vi "Initialize.vi"(8 "Error In":errorcluster, 9 "timeout in ms (-1)":i32=-1, 10 "WaitOnReply":bool, 11 "Payload":variant) -> (0 "error out":errorcluster, 2 "Reply":variant)   [LabVIEW 2017, in "ErrorHandler.lvlib"]
uses:
  ErrorHandler.lvlib
  States_FGVQ.ctl
  MessageData.ctl
  States_Module.ctl
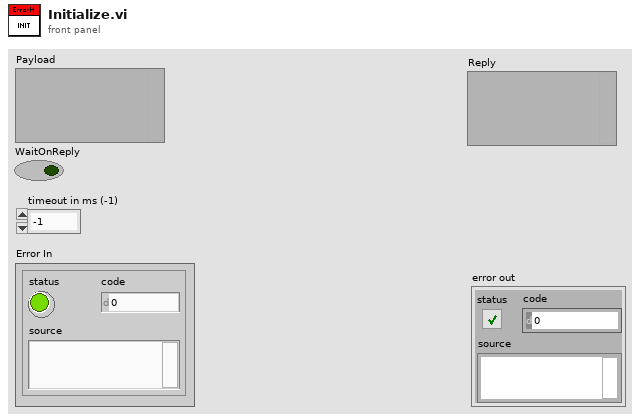
[diagram p1: front panel]
types:
  T1 = typedef "ErrorHandler.lvlib/States_Module.ctl" = enum16{"Error", "DoSomething", "Shutdown", "Initialize"}
  T2 = typedef "ErrorHandler.lvlib/MessageData.ctl" = cluster{"State":T1, "Payload":variant, "WaitOnReply":bool, "ReplyNotif":refnum<notifier>}
  T3 = typedef "ErrorHandler.lvlib/States_FGVQ.ctl" = enum16{"Get", "Shutdown", "Initialize"}
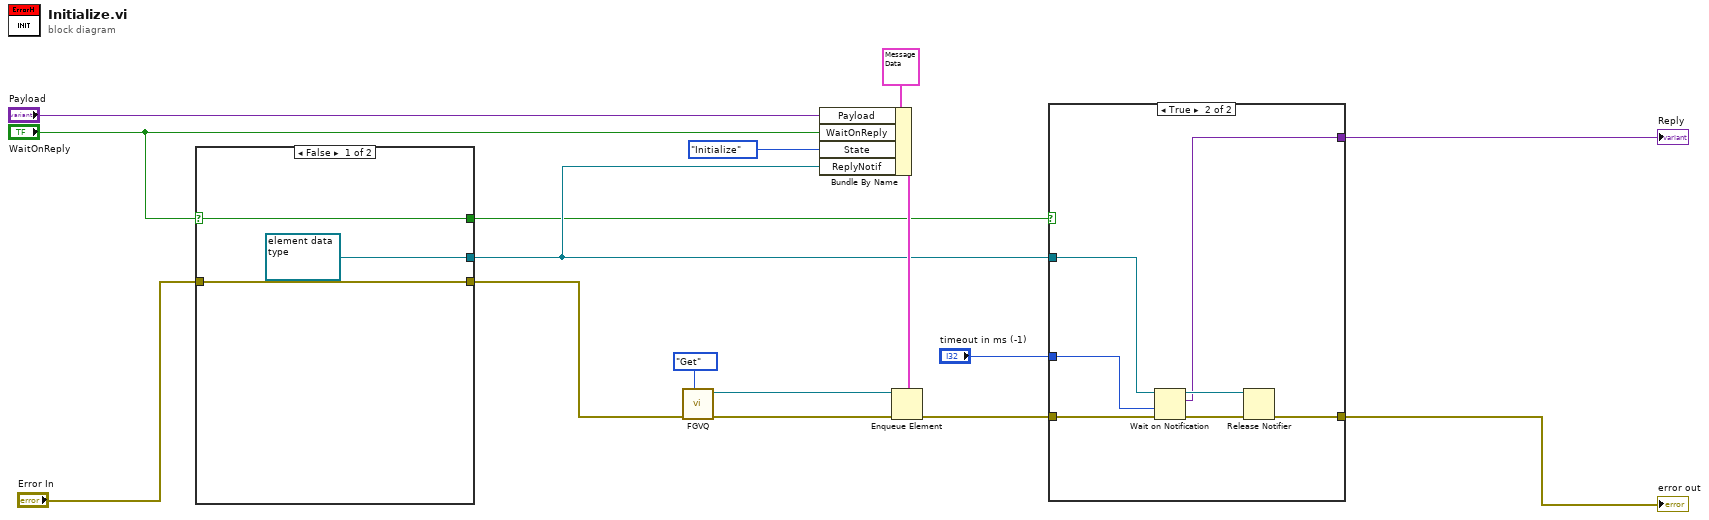
[diagram p0: block diagram]
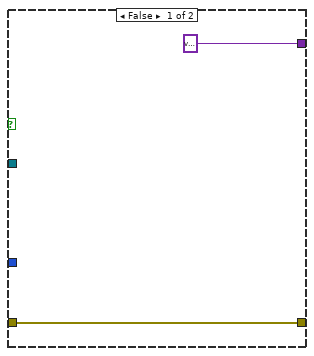
[diagram p2: hidden frame]
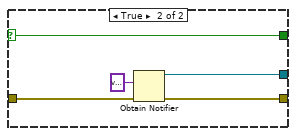
[diagram p3: hidden frame]
diagram:
  n1 = case shown="False" "WaitOnReply" {
    selector: "WaitOnReply" -> [w17 w20]
    tunnel: "Error In" -> [w19 w23]
    tunnel: [w19 w22] -> w7
    tunnel: [refnum<notifier> refnum ("notifier out") w21] -> w5
    tunnel: [w17 w20] -> w4
    frame False {
    }
    frame True {
      n2 = Obtain Notifier(notification data type=variant ("element data type"), error in (no error)=w23) -> (notifier out=w21:refnum<notifier>, error out=w22:errorcluster)  [unwired: 2 in, 1 out]
    }
  }
  n3 = call "FGVQ.vi"("State"=States_FGVQ."Get", "Error In"=w7) -> ("Error Out"=w15:errorcluster, "queue out"=w14:refnum<queue>)  [unwired: 8 in]
  n4 = Bundle By Name(cluster=T2 {"State"=enum."DoSomething", "Payload"=variant, "WaitOnReply"=TRUE, "ReplyNotif"=refnum} ("element"), "Payload"="Payload", "WaitOnReply"="WaitOnReply", "State"=States_Module."Initialize", "ReplyNotif"=w5) -> (w12:T2)
  n5 = Enqueue Element(queue=w14, element=w12, error in (no error)=w15) -> (error out=w6:errorcluster)  [unwired: 1 in, 2 out]
  n6 = case shown="True" w4 {
    tunnel: w6 -> [w26 w33]
    tunnel: w5 -> [_ w32]
    tunnel: "timeout in ms (-1)" -> [_ w31]
    tunnel: [w26 w29] -> w2
    tunnel: [variant ("element data type") w27] -> w1
    frame False {
    }
    frame True {
      n7 = Wait on Notification(notifier=w32, timeout in ms (-1)=w31, error in (no error)=w33) -> (notifier out=w28:refnum<notifier>, notification=w27:variant, error out=w30:errorcluster)  [unwired: 1 in, 1 out]
      n8 = Release Notifier(notifier=w28, error in (no error)=w30) -> (error out=w29:errorcluster)  [unwired: 1 in, 2 out]
    }
  }
  "error out" <- w2
  "Reply" <- w1
